vi "Connect.vi"(8 "error in":errorcluster, 11 "IF_XX in":refnum<class "IF_XX.lvclass">) -> (0 "error out":errorcluster, 3 "IF_XX out":refnum<class "IF_XX.lvclass">)   [LabVIEW 2019, in "IF_XX.lvlib" / "IF_XX.lvclass"]
doc: "This opens a TCPIP port to the IF-XX Power supply.\n\nThe example case shows a call to a scan for instruments step first. I'm not sure what the return values are from the scan operation, so this code has a risk for successful opening and closing."
uses:
  Library/IF_XX.lvclass
  C:/Users/Public/Documents/Development/builds/Instruments/Instruments.lvlibp/Library/Instruments.lvclass
  Library/IF_XX.lvclass/IF_XX.ctl
  builds/Instruments/Instruments.lvlibp/Accessors/Read Resource.vi
  builds/Instruments/PowerSupply.lvlibp/Library/PowerSupply.lvclass
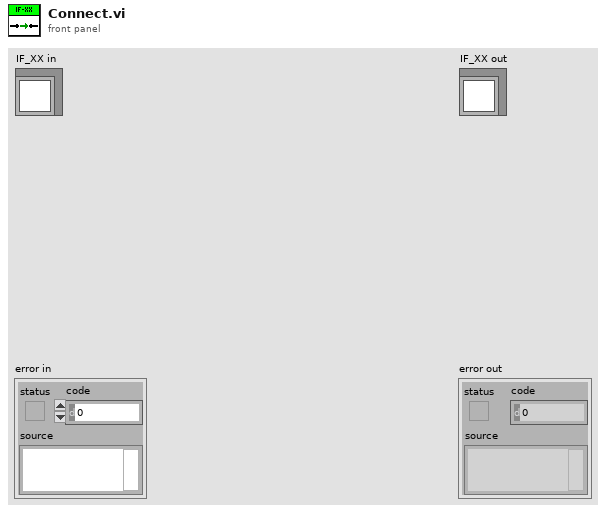
[diagram p1: front panel]
types:
  T1 = enum16{"All interfaces", "COM", "GPIB", "Ethernet", "COM + GPIB", "COM + Ethernet", "GPIB + Ethernet"}
  T2 = cluster{"IP range start":u8[], "IP range end":u8[], "Port":u16}
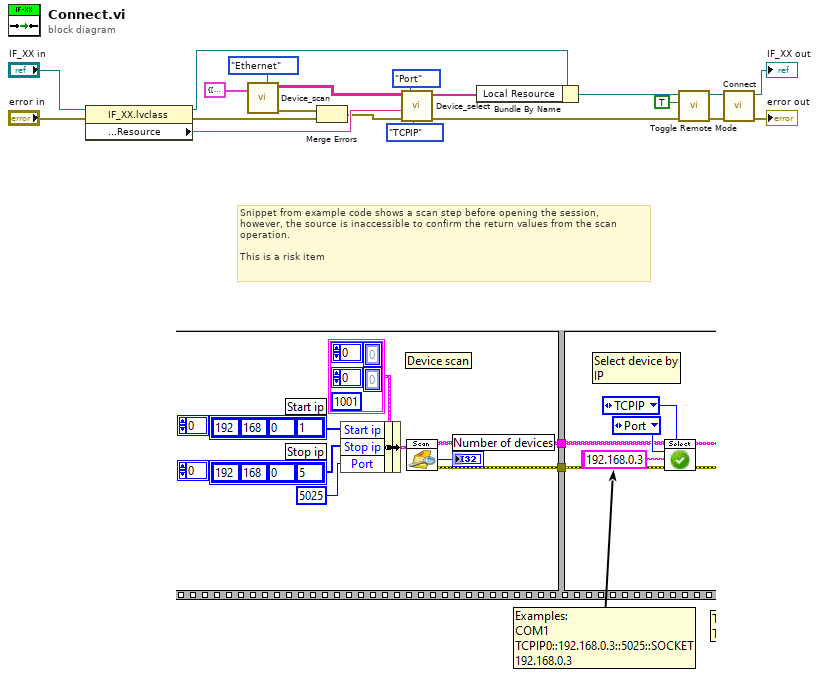
[diagram p0: block diagram]
diagram:
  # "Snippet from example code shows a scan step before opening the session,\nhowever, the source is inaccessible to confirm the return values from the scan\noperation.  \n\nThis is a risk item"
  n1 = property class="IF_XX.lvclass"(reference="IF_XX in", error in="error in") -> (reference out=w16:refnum<class "IF_XX.lvclass">, error out=w11:errorcluster, "Accessors:Configuration:Resource"=w13:string)
  n2 = call <instrlib>:"Device_scan.vi"("IP settings"=T2 {"IP range start"=[192, 168, 200, 10], "IP range end"=[192, 168, 200, 19], "Port"=5025}, "Scan mode"=T1."Ethernet") -> ("Device information array"=w4:string[][], "error out"=w2:errorcluster)  [unwired: 3 in, 1 out]
  n3 = Merge Errors(w2, w11) -> (w3:errorcluster)
  n4 = call <instrlib>:"Device_select.vi"("Reference"=enum16{"ASRL/COM", "GPIB", "TCPIP"}."TCPIP", "error in (no error)"=w3, "Number/Alias"=w13, "Open by"=enum16{"Serial number", "Port"}."Port", "Device information array"=w4) -> ("error out"=w9:errorcluster, "Device information"=w12:string[])  [unwired: 2 in]
  n5 = Bundle By Name(cluster=w16, "Local Resource"=w12) -> (w10:refnum<class "IF_XX.lvclass">)
  n6 = call "Toggle Remote Mode.vi"("error in (no error)"=w9, "Remote"=TRUE, "IF_XX in"=w10) -> ("error out"=w7:errorcluster, "IF_XX out"=w8:refnum<class "IF_XX.lvclass">)  [unwired: 7 in]
  n7 = call-parent "Connect.vi"("error in"=w7, "PowerSupply in"=w8) -> ("error out"=→"error out":errorcluster, "PowerSupply out"=→"IF_XX out":refnum<class "IF_XX.lvclass">)  [unwired: 8 in]
